vi "GetBoard.vi"(3 "Board in":refnum<class "Board_Game.lvclass">) -> (5 "Board":u32[][](array[colorbox]))   [LabVIEW 2021, in "Board_Game.lvclass"]
uses:
  Board_Game.lvclass
  Board_Game.lvclass/Board_Game.ctl
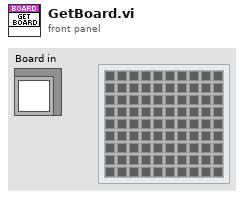
[diagram p1: front panel]
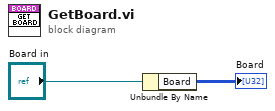
[diagram p0: block diagram]
diagram:
  n1 = Unbundle By Name("Board in") -> ("Board"=→"Board":u32[][])
